vi "Calcolo Hv12.vi"(8 "Q":dbl, 9 "l":dbl, 10 "d2":dbl, 11 "d1":dbl) -> (2 "Hv2":dbl, 3 "Hv1":dbl)   [LabVIEW 2019]
panel:
  # "Formula calcolo per perdita cono convergente (cono 1 in aspirazione, per angoli minori di 45°)\n\nK1=0,8*sin(teta/2)*(1-(d1^2/d2^2))\nteta=2*arctan(((d2-d1)/2)/lungh)\nv=Q(m3/sec)/sez(m2)\nsez=(d1/1000)^2*pigreco/4\nhv1=K1*(v^2/(2*g))\n\nK1=coefficente di perdita cono convergente\nteta=angolo apertura cono\nd1=diametro minore\nd2=diametro maggiore\nv=velocità caclolata su d1\nlungh=lunghezza cono\ng=9,80665"
  # "Formula calcolo per perdita cono divergente (cono 2 in mandata, per angoli minori di 45°)\n\nK2=2,6*sin(teta/2)*(1-(d1^2/d2^2))^2\nteta=2*arctan(((d2-d1)/2)/lungh)\nv=Q(m3/sec)/sez(m2)\nsez=(d1/1000)^2*pigreco/4\nhv2=K2*(v^2/(2*g))\n\nK2=coefficente di perdita cono divergente\nteta=angolo apertura cono\nd1=diametro minore\nd2=diametro maggiore\nv=velocità caclolata su d1 \nlungh=lunghezza cono"
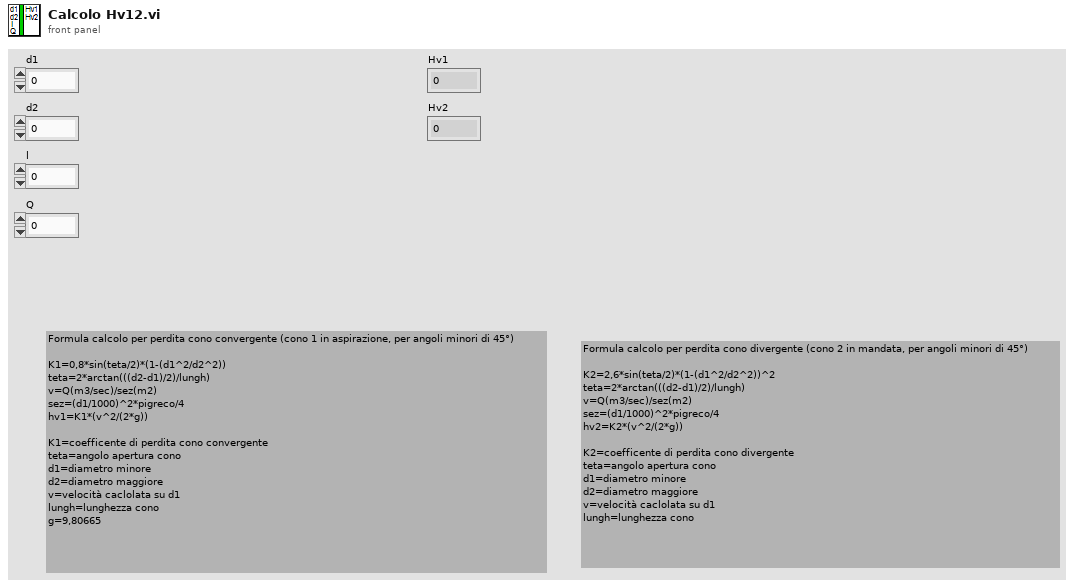
[diagram p1: front panel]
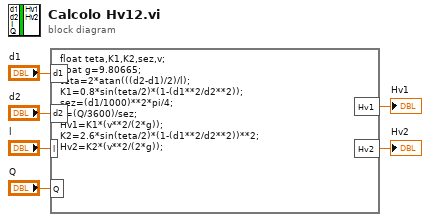
[diagram p0: block diagram]
diagram:
  n1 = formula code="float teta,K1,K2,sez,v;\nfloat g=9.80665;\nteta=2*atan(((d2-d1)/2)/l);\nK1=0.8*sin(teta/2)*(1-(d1**2/d2**2));\nsez=(d1/1000)**2*pi/4;\nv=(Q/3600)/sez;\nHv1=K1*(v**2/(2*g));\nK2=2.6*sin(teta/2)*(1-(d1**2/d2**2))**2;\nHv2=K2*(v**2/(2*g));"("d1"="d1", "d2"="d2", "l"="l", "Q"="Q") -> ("Hv1"=→"Hv1":dbl, "Hv2"=→"Hv2":dbl)
